vi "TestAPI.vi"(7 "LabVIEW Web Service Request":refnum<class "Web Request.lvclass">) -> ()   [LabVIEW 2025]
uses:
  <vilib>/wsapi/Web Request.lvclass
  VariabilaGlobala.vi
panel:
  # "Use the Web Service Request input terminal to call the VIs on the Web Services palette. Do not remove it from the connector pane unless you don't need access to the palette."
  # "Each additional control wired to the connector pane will be available as an input in the URL. To include an indicator in terminal-mode output (the default setting), it must also be wired to the connector pane."
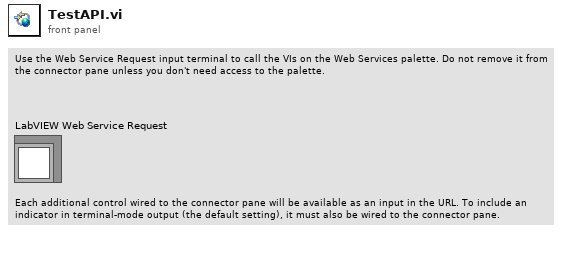
[diagram p1: front panel]
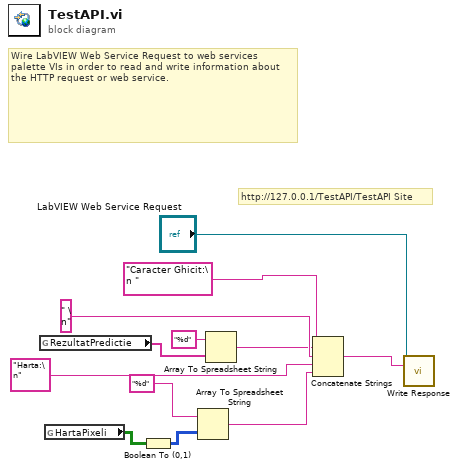
[diagram p0: block diagram]
diagram:
  # "http://127.0.0.1/TestAPI/TestAPI Site"
  # "Wire LabVIEW Web Service Request to web services palette VIs in order to read and write information about the HTTP request or web service."
  n1 = global read "VariabilaGlobala.vi" "RezultatPredictie"() -> (w3:string[])
  n2 = global read "VariabilaGlobala.vi" "HartaPixeli"() -> (w11:bool[][])
  n3 = Boolean To (0,1)(Boolean=w11) -> (0, 1=w10:i16[][])
  n4 = Array To Spreadsheet String(array=w10, 3:"%d" ("format string")) -> (spreadsheet string=w7:string)  [unwired: 1 in]
  n5 = Array To Spreadsheet String(array=w3, 3:"%d" ("format string")) -> (spreadsheet string=w2:string)  [unwired: 1 in]
  n6 = Concatenate Strings("Caracter Ghicit:\n " ("string"), w2, " \n" ("string"), "Harta:\n" ("string"), w7) -> (w8:string)
  n7 = call <vilib>:"Write Response.vi"("LabVIEW Web Service Request"="LabVIEW Web Service Request", "response string"=w8) -> ()  [unwired: 12 in, 2 out]
